vi "Load Yield Counts.vi"(8 "error in (no error)":errorcluster, 11 "Master in":refnum<class "Master.lvclass">) -> (0 "error out":errorcluster, 3 "Master out":refnum<class "Master.lvclass">)   [LabVIEW 2014]
uses:
  Programming Logic/Programing Logic.lvclass
  Master/Master.lvclass
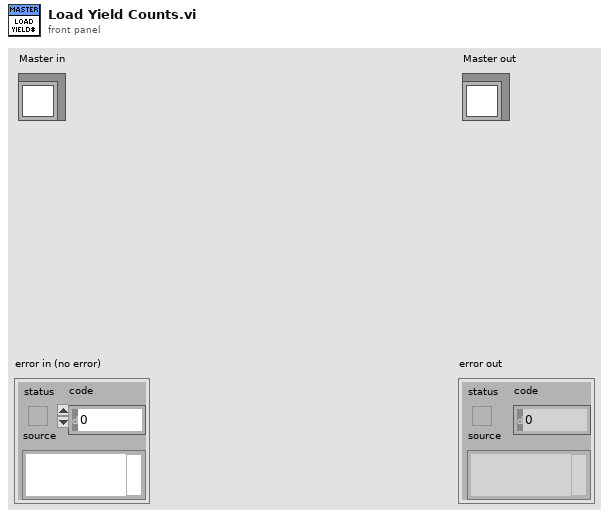
[diagram p1: front panel]
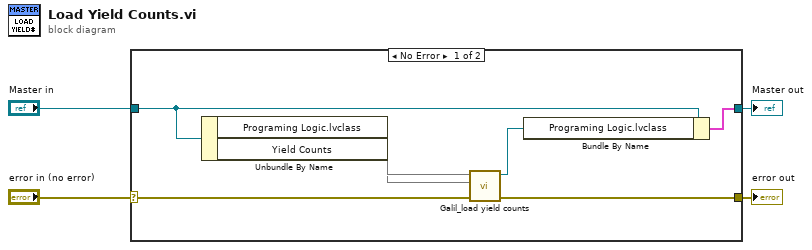
[diagram p0: block diagram]
diagram:
  n1 = case shown="No Error" "error in (no error)" {
    selector: "error in (no error)" -> [w6 w13]
    tunnel: [w5 w13] -> w3
    tunnel: [w9 w12] -> w1
    tunnel: "Master in" -> [w10 w12]
    frame No Error {
      n2 = Unbundle By Name(w10) -> ("Programing Logic.lvclass"=w11, "Yield Counts"=w7)
      n3 = call-dynamic "Galil_load yield counts.vi"("error in (no error)"=w6, "string"=w7, "Programing Logic in"=w11) -> ("error out"=w5:errorcluster, "Programing Logic out"=w8:refnum<class "Programing Logic.lvclass">)  [unwired: 7 in]
      n4 = Bundle By Name(cluster=w10, "Programing Logic.lvclass"=w8) -> (w9:cluster{})
    }
    frame Error {
    }
  }
  "error out" <- w3
  "Master out" <- w1
